vi "WritePSOC.vi"(7 "error in":errorcluster, 9 "write buffer":string, 10 "VISA resource name":refnum<visa-resource-name>="COM1") -> (0 "error out":errorcluster, 2 "return count":u32, 3 "VISA resource name out":refnum<visa-resource-name>)   [LabVIEW 2012]
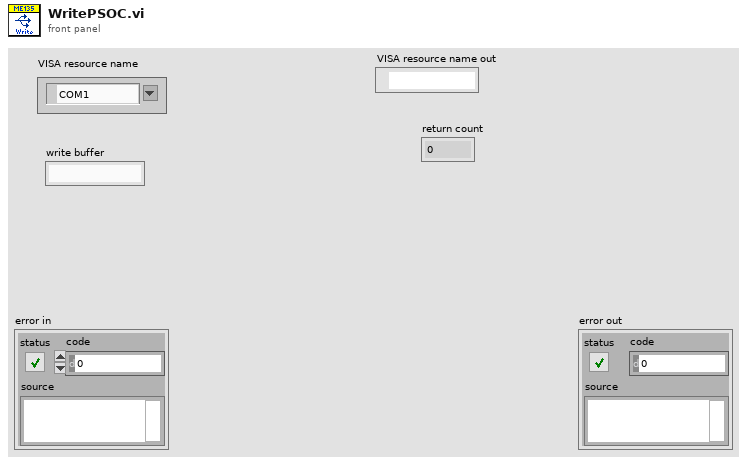
[diagram p1: front panel]
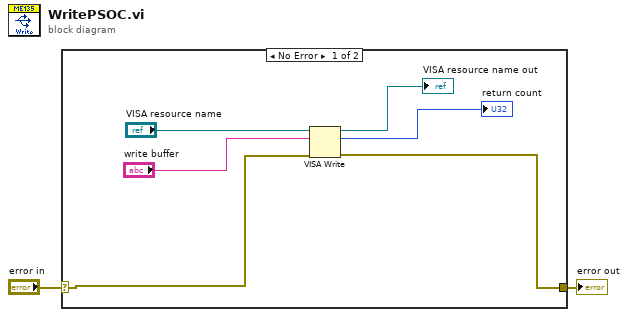
[diagram p0: block diagram]
diagram:
  n1 = case shown="No Error" "error in" {
    selector: "error in" -> [w8 w9]
    tunnel: [w7 w9] -> w1
    frame No Error {
      n2 = VISA Write(VISA resource name="VISA resource name", write buffer="write buffer", error in (no error)=w8) -> (VISA resource name out=→"VISA resource name out":refnum<visa-resource-name>, return count=→"return count":u32, error out=w7:errorcluster)
    }
    frame Error {
    }
  }
  "error out" <- w1
